vi "Create File Directories.vi"(8 "error in":errorcluster) -> (0 "error out":errorcluster)   [LabVIEW 2021]
doc: "Creates a folder for files to exist in."
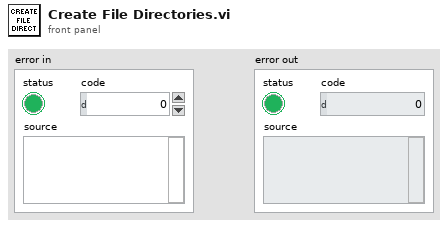
[diagram p1: front panel]
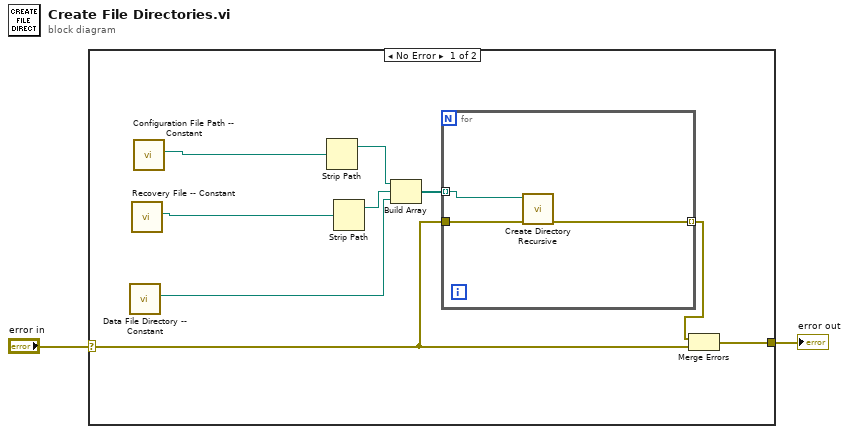
[diagram p0: block diagram]
diagram:
  n1 = case shown="No Error" "error in" {
    selector: "error in" -> [w4 w15]
    tunnel: [w5 w15] -> w1
    frame No Error {
      n2 = call "Data File Directory -- Constant.vi"() -> ("Data File Directory"=w9:path)  [unwired: 11 in]
      n3 = call "Recovery File -- Constant.vi"() -> ("Recovery File Path"=w10:path)  [unwired: 11 in]
      n4 = call "Configuration File Path -- Constant.vi"() -> ("Configuration File Path"=w11:path)  [unwired: 11 in]
      n5 = Strip Path(path=w11) -> (stripped path=w7:path)  [unwired: 1 out]
      n6 = Strip Path(path=w10) -> (stripped path=w8:path)  [unwired: 1 out]
      n7 = Build Array(w7, w8, w9) -> (w6:path[])
      n8 = for {
        tunnel: w6 -> [w14] mode=indexing
        tunnel: [w13] -> w3 mode=indexing
        tunnel: w4 -> [w12]
        n9 = call <vilib>:"Create Directory Recursive.vi"("error in (no error)"=w12, "directory"=w14) -> ("error out"=w13:errorcluster)  [unwired: 3 in, 2 out]
      }
      n10 = Merge Errors(w3, w4) -> (w5:errorcluster)
    }
    frame Error {
    }
  }
  "error out" <- w1
